vi "All Values.vi"(8 "error in (no error)":errorcluster, 11 "Group BOOL in":refnum<class "Group BOOL.lvclass">) -> (0 "error out":errorcluster, 1 "Timestamp":dbl[](array[numeric]), 2 "Scaled":bool[](array[boolean]), 3 "Group BOOL out":refnum<class "Group BOOL.lvclass">, 4 "Raw":bool[](array[boolean]))   [LabVIEW 2020, in "Vecto.lvlib" / "Group BOOL.lvclass"]
uses:
  Group BOOL.lvclass
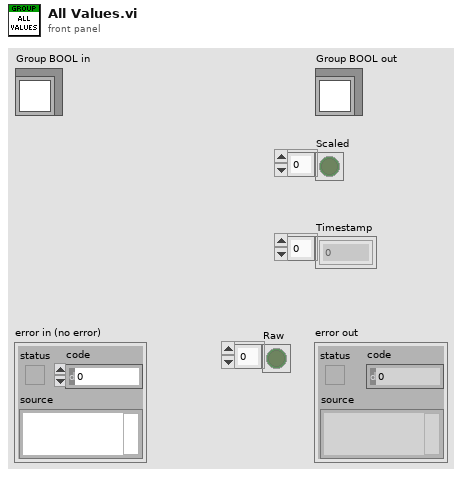
[diagram p1: front panel]
types:
  T1 = typedef "Vecto.lvlib/Group BOOL.lvclass/Ref.ctl" = cluster{"Scaled":bool[], "Timestamp":dbl[], "Raw":bool[]}
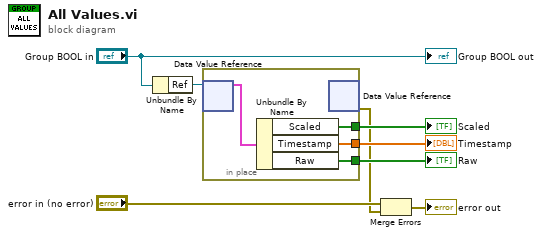
[diagram p0: block diagram]
diagram:
  n1 = Unbundle By Name("Group BOOL in") -> ("Ref"=w7:refnum<data-value>)
  n2 = in-place {
    in-place-border: [w11] -> w5
    in-place-border: [w10] -> w4
    in-place-border: [w9] -> w3
    n3 = in-place-dvr #1(w7) -> (w12:T1)  [unwired: 1 out]
    n4 = Unbundle By Name(w12) -> ("Scaled"=w11:bool[], "Timestamp"=w10:dbl[], "Raw"=w9:bool[])
    n5 = in-place-dvr #1() -> (w1:errorcluster)  [unwired: 1 in, 1 out]
  }
  "Scaled" <- w5
  "Timestamp" <- w4
  "Raw" <- w3
  n6 = Merge Errors("error in (no error)", w1) -> (→"error out":errorcluster)
  "Group BOOL out" <- "Group BOOL in"
